vi "Save Result.vi"(6 "Data":string[][](array[string]), 7 "Table":refnum<vi>, 8 "error in (no error)":errorcluster, 9 "布尔":bool, 10 "ProductID":string, 11 "strXMLResultText":string) -> (0 "error out":errorcluster, 1 "结果字符串":string, 2 "Error Code":i64, 3 "Operation Success":bool)   [LabVIEW 2017]
panel:
  in  "FFTester._Tester":refnum<k7>
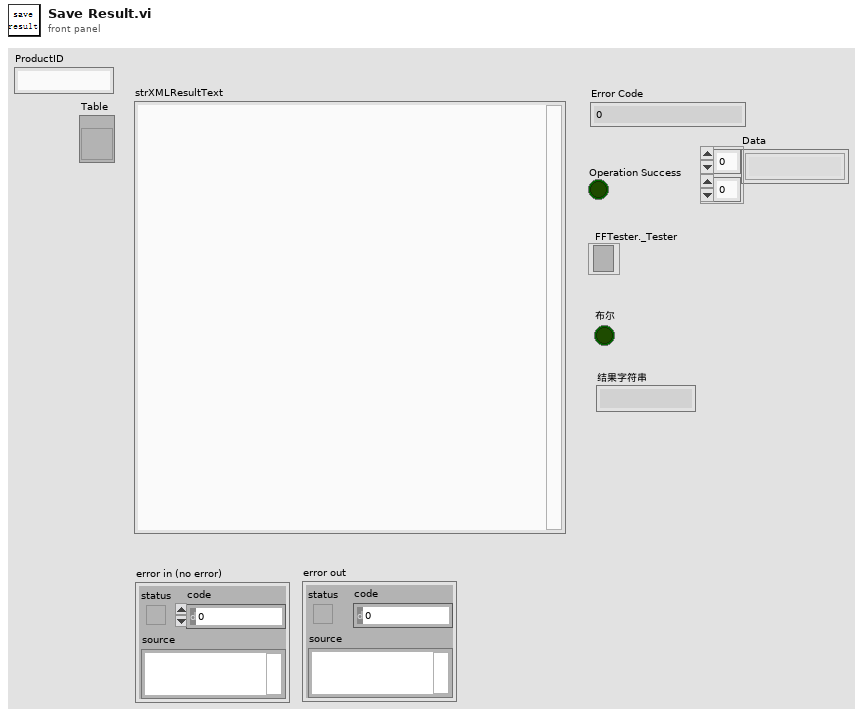
[diagram p1: front panel]
types:
  T1 = enum16{"open", "replace", "create", "open or create", "replace or create", "replace or create with confirmation"}
  T2 = typedef "TesterInfo.ctl" = cluster{"Station Name":string, "Station Code":string, "ES NO.":string, "Tester ID":string, "PassMark Revision":string, "Rig ID":string, "Deamon_vision":string, "Project Name":string, "FFTesterPath":path, "Enable_User":bool, "Mode":enum16{"682"}, "MES":bool}
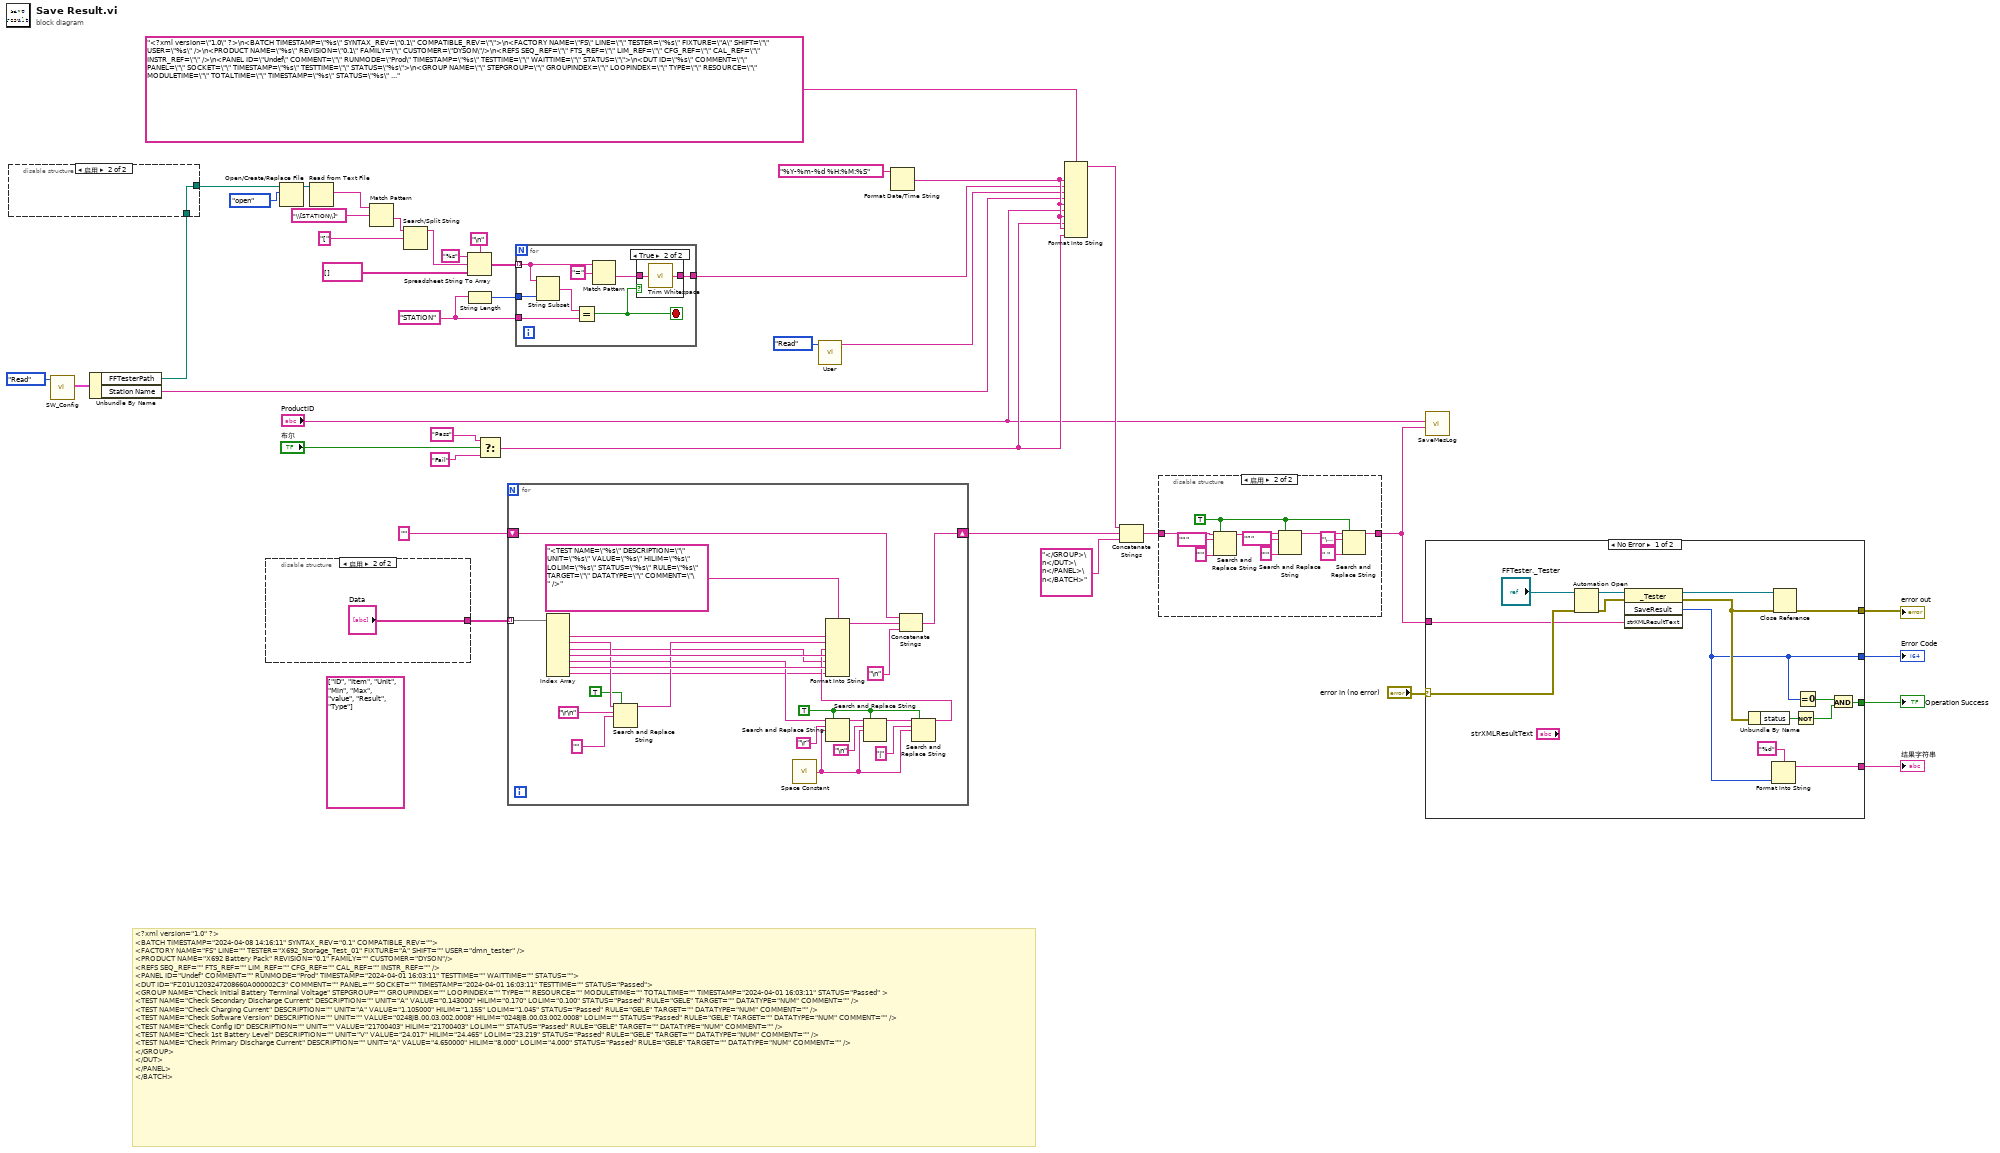
[diagram p0: block diagram]
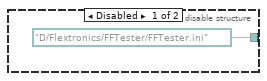
[diagram p3: hidden frame]
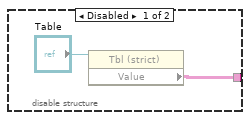
[diagram p4: hidden frame]
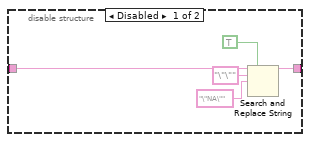
[diagram p5: hidden frame]
diagram:
  (unwired) string[] ["ID", "Item", "Unit", "Min", "Max", "value", "Result", "Type"] ("列首字符串[]")
  w5 = "STATION"
  # "<?xml version=\"1.0\" ?>\n<BATCH TIMESTAMP=\"2024-04-08 14:16:11\" SYNTAX_REV=\"0.1\" COMPATIBLE_REV=\"\">\n<FACTORY NAME=\"FS\" LINE=\"\" TESTER=\"X692_Storage_Test_01\" FIXTURE=\"A\" SHIFT=\"\" USER=\"dmn_tester\" />\n<PRODUCT NAME=\"X692 Battery Pack\" REVISION=\"0.1\" FAMILY=\"\" CUSTOMER=\"DYSON\"/>\n<REFS SEQ_REF=\"\" FTS_REF=\"\" LIM_REF=\"\" CFG_REF=\"\" CAL_REF=\"\" INSTR_REF=\"\" />\n<PANEL ID=\"Undef\" COMMENT=\"\" RUNMODE=\"Prod\" TIMESTAMP=\"2024-04-01 16:03:11\" TESTTIME=\"\" WAITTIME=\"\" STATUS=\"\">\n<DUT ID=\"FZ01U1203247208660A000002C3\" COMMENT=\"\" PANEL=\"\" SOCKET=\"\" TIMESTAMP=\"2024-04-01 16:03:11\" TESTTIME=\"\" STATUS=\"Passed\">\n<GROUP NAME=\"Check Initial Battery Terminal Voltage\" STEPGROUP=\"\" GROUPINDEX=\"\" LOOPINDEX=\"\" TYPE=\"\" RESOURCE=\"\" MODULETIME=\"\" TOTALTIME=\"\" TIMESTAMP=\"2024-04-01 16:03:11\" STATUS=\"Passed\" >\n<TEST NAME=\"Check Secondary Discharge Current\" DESCRIPTION=\"\" UNIT=\"A\" VALUE=\"0.143000\" HILIM=\"0.170\" LOLIM=\"0.100\" STATUS=\"Passed\" RULE=\"GELE\" TARGET=\"\" DATATYPE=\"NUM\" COMMENT=\"\" />\n<TEST NAME=\"Check Charging Current\" DESCRIPTION=\"\" UNIT=\"A\" VALUE=\"1.105000\" HILIM=\"1.155\" LOLIM=\"1.045\" STATUS=\"Passed\" RULE=\"GELE\" TARGET=\"\" DATATYPE=\"NUM\" COMMENT=\"\" />\n<TEST NAME=\"Check Software Version\" DESCRIPTION=\"\" UNIT=\"\" VALUE=\"0248JB.00.03.002.0008\" HILIM=\"0248JB.00.03.002.0008\" LOLIM=\"\" STATUS=\"Passed\" RULE=\"GELE\" TARGET=\"\" DATATYPE=\"NUM\" COMMENT=\"\" />\n<TEST NAME=\"Check Config ID\" DESCRIPTION=\"\" UNIT=\"\" VALUE=\"21700403\" HILIM=\"21700403\" LOLIM=\"\" STATUS=\"Passed\" RULE=\"GELE\" TARGET=\"\" DATATYPE=\"NUM\" COMMENT=\"\" />\n<TEST NAME=\"Check 1st Battery Level\" DESCRIPTION=\"\" UNIT=\"V\" VALUE=\"24.017\" HILIM=\"24.465\" LOLIM=\"23.219\" STATUS=\"Passed\" RULE=\"GELE\" TARGET=\"\" DATATYPE=\"NUM\" COMMENT=\"\" />\n<TEST NAME=\"Check Primary Discharge Current\" DESCRIPTION=\"\" UNIT=\"A\" VALUE=\"4.650000\" HILIM=\"8.000\" LOLIM=\"4.000\" STATUS=\"Passed\" RULE=\"GELE\" TARGET=\"\" DATATYPE=\"NUM\" COMMENT=\"\" />\n</GROUP>\n</DUT>\n</PANEL>\n</BATCH>"
  n1 = call "SW_Config.vi"("Step"=enum16{"Initial", "Write", "Read"}."Read") -> ("SW Config out"=w1:T2)  [unwired: 9 in, 1 out]
  n2 = Unbundle By Name(w1) -> ("FFTesterPath"=w18:path, "Station Name"=w17:string)
  n3 = disable-structure shown="启用" {
    disable-tunnel: [path "D:/Flextronics/FFTester/FFTester.ini" ("路径") w43] -> w3
    disable-tunnel: w18 -> [_ w43]
    frame Disabled {
    }
    frame Enabled {
    }
  }
  n4 = disable-structure shown="启用" {
    disable-tunnel: [w44 "Data"] -> w24
    frame Disabled {
      n5 = property class="Tbl (strict)"(reference="Table") -> ("Value"=w44:string[][])  [unwired: 1 in, 2 out]
    }
    frame Enabled {
    }
  }
  n6 = Open/Create/Replace File(file path (use dialog)=w3, operation (0:open)=T1."open" ("操作(0:open)")) -> (refnum out=w16:refnum<file>)  [unwired: 4 in, 2 out]
  n7 = Read from Text File(file (use dialog)=w16) -> (text=w11:string)  [unwired: 3 in, 3 out]
  n8 = Match Pattern(string=w11, regular expression="\\[STATION\\]") -> (after substring=w12:string)  [unwired: 1 in, 3 out]
  n9 = Search/Split String(string=w12, search string/char (-)="[") -> (substring before match=w9:string)  [unwired: 1 in, 2 out]
  n10 = Spreadsheet String To Array(delimiter (Tab)="\n" ("分隔符(Tab)"), format string="%s" ("格式字符串"), spreadsheet string=w9, array type (2D Dbl)=string[] []) -> (array=w6:string[])
  n11 = String Length(string=w5) -> (length=w4:i32)
  n12 = Select(t="Pass", s="布尔", f="Fail") -> (s? t:f=w28:string)
  n13 = for {
    tunnel: w24 -> [w71] mode=indexing
    shift-right: [w63] -> w22
    shift-left: "" -> [w64]
    w49 = TRUE ("替换全部？(F)")
    n14 = Index Array(array=w71) -> (element #2=w69:string, element #3=w62:string, element #4=w48:string, element #5=w68:string, element #6=w54:string, element #7=w67:string, element #8=w47:string)  [unwired: 8 in, 1 out]
    n15 = Search and Replace String(replace all?=TRUE, input string=w62, search string="\r\n", replace string="") -> (result string=w58:string)  [unwired: 4 in, 3 out]
    n16 = call <vilib>:"Space Constant.vi"() -> ("String"=w50:string)
    n17 = Search and Replace String(replace all?=w49, input string=w54, search string="\r", replace string=w50) -> (result string=w57:string)  [unwired: 4 in, 3 out]
    n18 = Search and Replace String(replace all?=w49, input string=w57, search string="\n", replace string=w50) -> (result string=w53:string)  [unwired: 4 in, 3 out]
    n19 = Search and Replace String(replace all?=w49, input string=w53, search string="|", replace string=w50) -> (result string=w52:string)  [unwired: 4 in, 3 out]
    n20 = Format Into String(format string="<TEST NAME=\"%s\" DESCRIPTION=\"\" UNIT=\"%s\" VALUE=\"%s\" HILIM=\"%s\" LOLIM=\"%s\" STATUS=\"%s\" RULE=\"%s\" TARGET=\"\" DATATYPE=\"\" COMMENT=\"\" />", w69, w58, w52, w68, w48, w67, w47) -> (resulting string=w66:string)  [unwired: 2 in, 1 out]
    n21 = Concatenate Strings(w64, w66, "\n") -> (w63:string)
  }
  n22 = for {
    tunnel: w6 -> [w76] mode=indexing
    tunnel: w5 -> [w77]
    tunnel: w4 -> [w79]
    tunnel: [w73] -> w2
    stop <- w72 stop-if-true
    n23 = String Subset(string=w76, length (rest)=w79) -> (substring=w78:string)  [unwired: 1 in]
    n24 = Equal?(x=w78, y=w77) -> (x = y?=w72:bool)
    n25 = Match Pattern(string=w76, regular expression="=" ("正则表达式")) -> (after substring=w74:string)  [unwired: 1 in, 3 out]
    n26 = case shown="True" w72 {
      tunnel: w74 -> [_ w81]
      tunnel: [_ w80] -> w73
      frame False {
      }
      frame True {
        n27 = call <vilib>:"Trim Whitespace.vi"("string"=w81) -> ("trimmed string"=w80:string)  [unwired: 1 in]
      }
    }
  }
  n28 = call "User.vi"("Step"=enum16{"Initial", "Write", "Read"}."Read") -> ("User out"=w20:string)  [unwired: 9 in, 1 out]
  n29 = Format Date/Time String(time format string (%c)="%Y-%m-%d %H:%M:%S" ("时间格式字符串(%c)")) -> (date/time string=w29:string)  [unwired: 2 in]
  n30 = Format Into String(format string="<?xml version=\"1.0\" ?>\n<BATCH TIMESTAMP=\"%s\" SYNTAX_REV=\"0.1\" COMPATIBLE_REV=\"\">\n<FACTORY NAME=\"FS\" LINE=\"\" TESTER=\"%s\" FIXTURE=\"A\" SHIFT=\"\" USER=\"%s\" />\n<PRODUCT NAME=\"%s\" REVISION=\"0.1\" FAMILY=\"\" CUSTOMER=\"DYSON\"/>\n<REFS SEQ_REF=\"\" FTS_REF=\"\" LIM_REF=\"\" CFG_REF=\"\" CAL_REF=\"\" INSTR_REF=\"\" />\n<PANEL ID=\"Undef\" COMMENT=\"\" RUNMODE=\"Prod\" TIMESTAMP=\"%s\" TESTTIME=\"\" WAITTIME=\"\" STATUS=\"\">\n<DUT ID=\"%s\" COMMENT=\"\" PANEL=\"\" SOCKET=\"\" TIMESTAMP=\"%s\" TESTTIME=\"\" STATUS=\"%s\">\n<GROUP NAME=\"\" STEPGROUP=\"\" GROUPINDEX=\"\" LOOPINDEX=\"\" TYPE=\"\" RESOURCE=\"\" MODULETIME=\"\" TOTALTIME=\"\" TIMESTAMP=\"%s\" STATUS=\"%s\" >\n", w29, w2, w20, w17, w29, "ProductID", w29, w28, w29, w28) -> (resulting string=w34:string)  [unwired: 2 in, 1 out]
  n31 = Concatenate Strings(w34, w22, "</GROUP>\n</DUT>\n</PANEL>\n</BATCH>") -> (w33:string)
  n32 = disable-structure shown="启用" {
    disable-tunnel: [w86 w88] -> w25
    disable-tunnel: w33 -> [w85 w92]
    frame Disabled {
      n33 = Search and Replace String(replace all?=TRUE ("替换全部？(F)"), input string=w85, search string="\"\"" ("搜索字符串"), replace string="\"NA\"" ("搜索字符串")) -> (result string=w86:string)  [unwired: 4 in, 3 out]
    }
    frame Enabled {
      w87 = TRUE ("替换全部？(F)")
      n34 = Search and Replace String(replace all?=w87, input string=w92, search string="“" ("搜索字符串"), replace string="'" ("替换字符串(\"\")")) -> (result string=w93:string)  [unwired: 4 in, 3 out]
      n35 = Search and Replace String(replace all?=w87, input string=w93, search string="”" ("搜索字符串"), replace string="'" ("替换字符串(\"\")")) -> (result string=w89:string)  [unwired: 4 in, 3 out]
      n36 = Search and Replace String(replace all?=w87, input string=w89, search string="\u0000" ("搜索字符串"), replace string=" " ("替换字符串(\"\")")) -> (result string=w88:string)  [unwired: 4 in, 3 out]
    }
  }
  n37 = call "SaveMesLog.vi"("String"=w25, "SN"="ProductID") -> ()  [unwired: 10 in]
  n38 = case shown="No Error" "error in (no error)" {
    selector: "error in (no error)" -> [w105 w113]
    tunnel: [w112 w113] -> w41
    tunnel: [w99 _] -> w39
    tunnel: [w108 _] -> w38
    tunnel: w25 -> [w101 _]
    tunnel: [w98 _] -> w27
    frame No Error {
      n39 = Automation Open(error in (no error)=w105, Automation Refnum="FFTester._Tester") -> (Automation Refnum=w107:refnum<k7>, error out=w104:errorcluster)  [unwired: 2 in]
      n40 = invoke on="调用节点" class="_Tester" method="SaveResult"(reference=w107, error in=w104, "strXMLResultText"=w101) -> (reference out=w102:refnum<k7>, error out=w103:errorcluster, "SaveResult"=w99:i32)  [unwired: 1 in, 1 out]
      n41 = Unbundle By Name(w103) -> ("status"=w111:bool)
      n42 = Format Into String(format string="%d" ("格式字符串"), w99) -> (resulting string=w98:string)  [unwired: 2 in, 1 out]
      n43 = Close Reference(reference=w102, error in (no error)=w103) -> (error out=w112:errorcluster)
      n44 = Not(x=w111) -> (.not. x?=w109:bool)
      n45 = Equal To 0?(x=w99) -> (x = 0?=w110:bool)
      n46 = And(x=w110, y=w109) -> (x .and. y?=w108:bool)
    }
    frame Error {
    }
  }
  "error out" <- w41
  "Error Code" <- w39
  "Operation Success" <- w38
  "结果字符串" <- w27
